vi "Arrow_Notifier_Begin.vi"   [LabVIEW 2020]
uses:
  Subsystems/Arrow/Arrow_Control_States.ctl
  Subsystems/Arrow/Arrow_Cluster.ctl
  Globals/Arrow_Globals.vi
types:
  T1 = typedef "Arrow_Cluster.ctl" = cluster{"Control_States":T2, "Manual_Arrow":dbl}
  T2 = typedef "Arrow_Control_States.ctl" = enum16{"No-Op", "Manual_Control", "GoToAngle"}
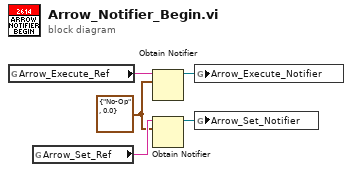
[diagram p0: block diagram]
diagram:
  w1 = T1 {"Control_States"=enum."No-Op", "Manual_Arrow"=0.0}
  n1 = global read "Arrow_Globals.vi" "Arrow_Execute_Ref"() -> (w2:string)
  n2 = global read "Arrow_Globals.vi" "Arrow_Set_Ref"() -> (w3:string)
  n3 = Obtain Notifier(name (unnamed)=w2, notification data type=w1) -> (notifier out=w5:refnum<notifier>)  [unwired: 2 in, 2 out]
  n4 = Obtain Notifier(name (unnamed)=w3, notification data type=w1) -> (notifier out=w4:refnum<notifier>)  [unwired: 2 in, 2 out]
  n5 = global write "Arrow_Globals.vi" "Arrow_Execute_Notifier"(w5) -> ()
  n6 = global write "Arrow_Globals.vi" "Arrow_Set_Notifier"(w4) -> ()
